vi "RT Driver VI.vi"(7 "Operation":T1, 11 "Device Reference in":T2 format="%.0x") -> (0 "Error Code":i32)   [LabVIEW 2014, in "SLSC configuration Engine.lvlib"]
uses:
  SLSC configuration Engine.lvlib
  <vilib>/NI Veristand/Custom Device API/Custom Device Item Ref.ctl
  <vilib>/NI Veristand/Custom Device API/Hardware Interface Driver VI Operation.ctl
  Type Defs/RT data.ctl
  Type Defs/RT Engine Refs.ctl
  Shared/Type Defs/RT IDs.ctl
  Shared/SPI Utility/Slot #.ctl
  Shared/MCP23S17/Chip Address.ctl
  <vilib>/NI Veristand/Custom Device API/Block Data Reference.ctl
  <vilib>/NI Veristand/Custom Device API/Data Reference.ctl
  <vilib>/FPGAPlugInAG/Dynamic/niLvFpga_Close_Dynamic.vi
  <vilib>/rvi/interface/nirviCloseFPGA/nirviCloseFPGA.xnode
  Shared/SLSC configuration Shared.lvlib
  <vilib>/NI Veristand/Custom Device API/Custom Device API.lvlib
  <vilib>/NI Veristand/Custom Device Tools/Custom Device Utility Library/Custom Device Utility Library.lvlib
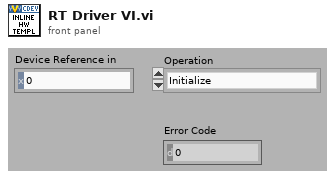
[diagram p1: front panel]
types:
  T1 = typedef "Custom Device API.lvlib/Hardware Interface Driver VI Operation.ctl" = enum16{"Initialize", "Start", "Read Data from HW", "Write Data to HW", "Close"}
  T2 = typedef "Custom Device API.lvlib/Custom Device Item Ref.ctl" = u64
  T3 = typedef "SLSC configuration Engine.lvlib/RT data.ctl" = cluster{"Bitfile ref":refnum<k20>, "Device Error":errorcluster, "FIU Engine Refs":T4, "DMA FIFO ref":refnum<k20>, "Battery Switch Engine Refs":T4, "Wheel Speed Sensor Engine Refs":T4, "Resistor Engine Refs":T4, "Current Sense Engine Refs":T4, "Device Name":string, "LED Engine Refs":T4, "DIO Engine Refs":T4}
  T4 = typedef "SLSC configuration Engine.lvlib/RT Engine Refs.ctl" = cluster{"RT IDs":T5[], "RT Block Data Refs":T8[], "RT Channel Values":dbl[]}
  T5 = typedef "SLSC configuration Shared.lvlib/RT IDs.ctl" = cluster{"Rack #":u8, "Slot #":T6, "Chip Address (A2 A1 A0)":T7}
  T6 = typedef "SLSC configuration Shared.lvlib/Slot #.ctl" = u8
  T7 = typedef "SLSC configuration Shared.lvlib/Chip Address.ctl" = u8
  T8 = typedef "Custom Device API.lvlib/Block Data Reference.ctl" = cluster{"Data Reference":T9, "Offset":i32, "Length":i32}
  T9 = typedef "Custom Device API.lvlib/Data Reference.ctl" = i32
  T10 = typedef "Custom Device API.lvlib/Custom Device Item Info.ctl" = cluster{"Name":string, "Is Channel":bool, "GUID":string, "Is Waveform":bool}
  T11 = typedef "SLSC configuration Shared.lvlib/SLSC compiled.ctl" = cluster{"FIU Engine Data":T12, "Battery Switch Engine Data":T12, "Wheel Speed Sensor Engine Data":T12, "Resistor Engine Data":T12, "Current Sense Engine Data":T12, "LED Engine Data":T12, "DIO Engine Data":T12}
  T12 = typedef "SLSC configuration Shared.lvlib/RT Engine Data.ctl" = cluster{"RT IDs":T5[], "Ordered Channels":T2[]}
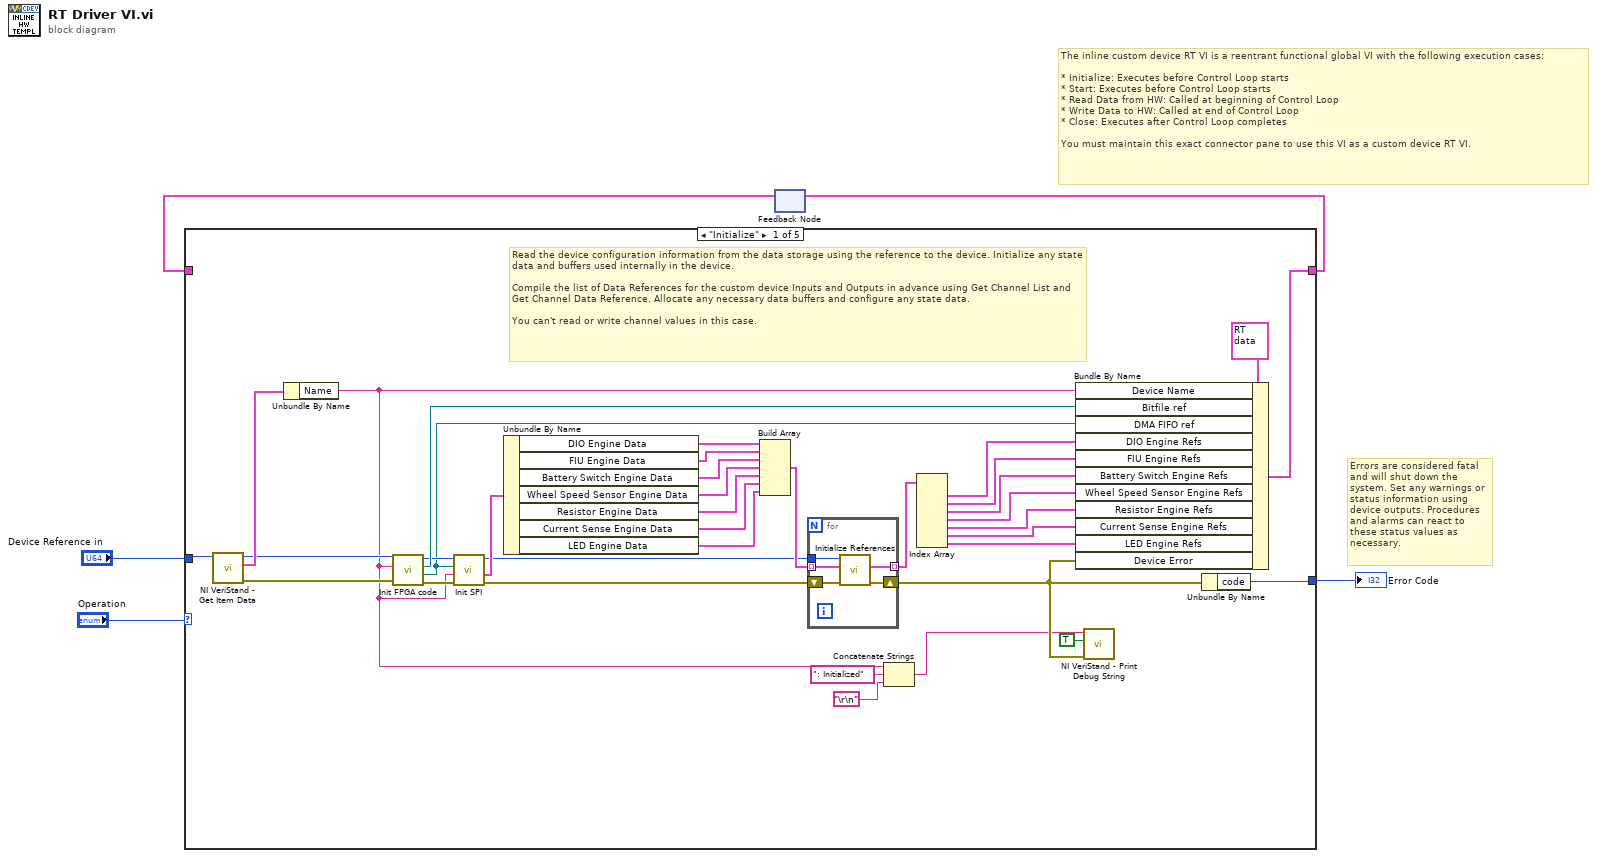
[diagram p0: block diagram]
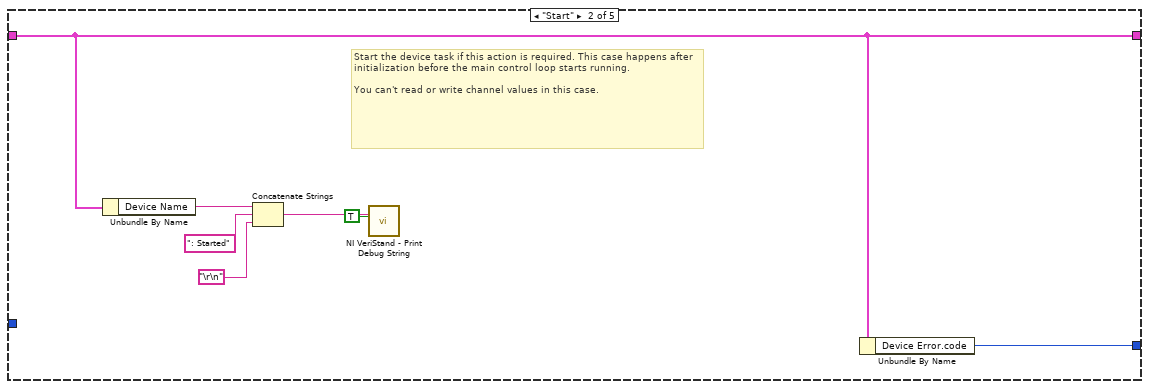
[diagram p2: hidden frame]
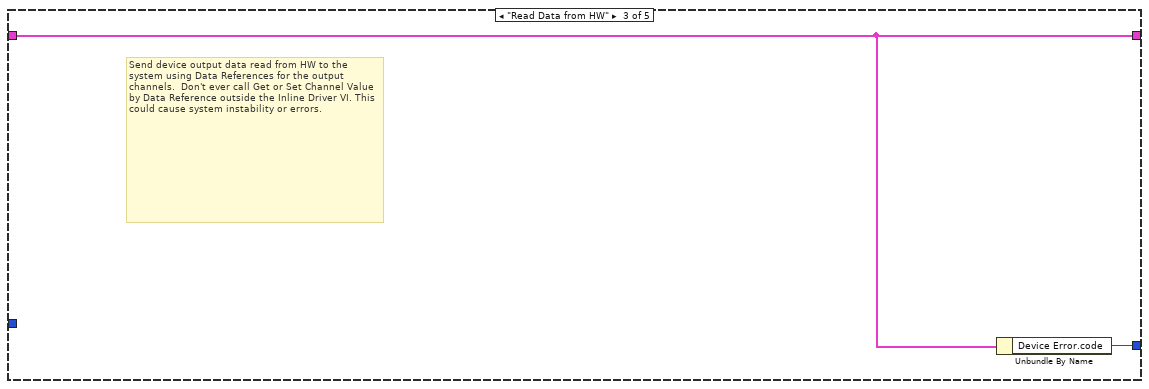
[diagram p3: hidden frame]
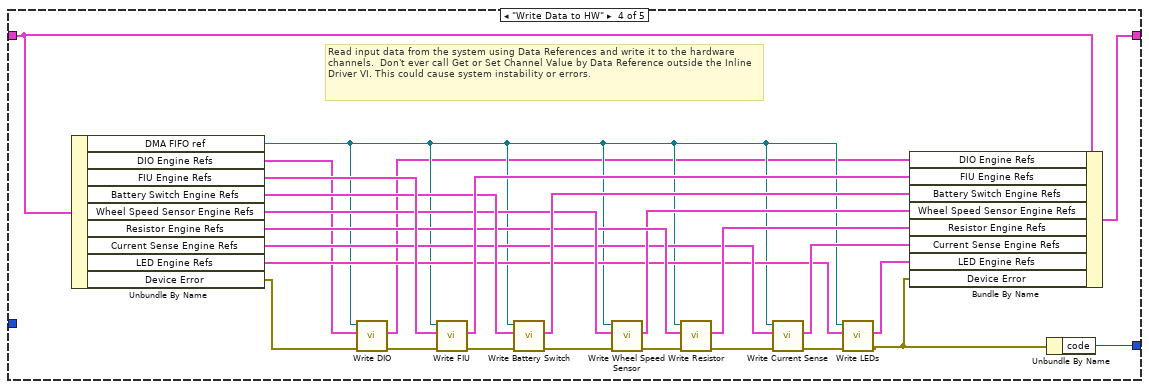
[diagram p4: hidden frame]
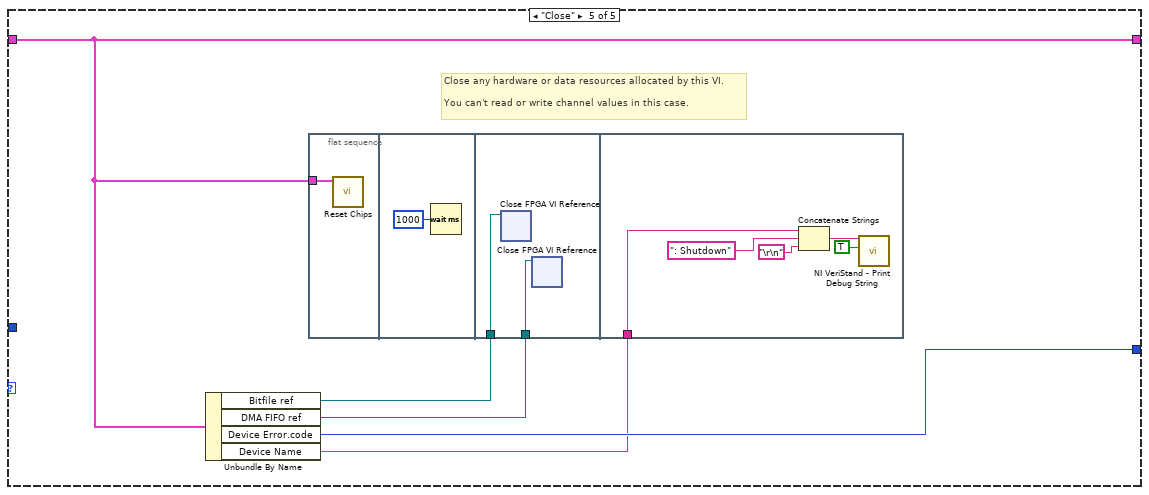
[diagram p5: hidden frame]
diagram:
  # "Errors are considered fatal and will shut down the system. Set any warnings or status information using device outputs. Procedures and alarms can react to these status values as necessary."
  # "The inline custom device RT VI is a reentrant functional global VI with the following execution cases:\n\n* Initialize: Executes before Control Loop starts\n* Start: Executes before Control Loop starts\n* Read Data from HW: Called at beginning of Control Loop\n* Write Data to HW: Called at end of Control Loop\n* Close: Executes after Control Loop completes\n\nYou must maintain this exact connector pane to use this VI as a custom device RT VI."
  n1 = feedback #1() -> (w3:T3)  [unwired: 1 out]
  n2 = case shown="\"Initialize\"" "Operation" {
    tunnel: [w41 w52 w54 w80 w85] -> w4
    tunnel: w3 -> [_ w52 w54 w81 w85]
    tunnel: "Device Reference in" -> [w21 _ _ _ _]
    tunnel: [w40 w53 w55 w79 w86] -> w1
    frame "Initialize" {
      # "Read the device configuration information from the data storage using the reference to the device. Initialize any state data and buffers used internally in the device.\n\nCompile the list of Data References for the custom device Inputs and Outputs in advance using Get Channel List and Get Channel Data Reference. Allocate any necessary data buffers and configure any state data.\n\nYou can't read or write channel values in this case."
      n3 = call <vilib>:"NI VeriStand - Get Item Data.vi"("Item Ref in"=w21) -> ("error out"=w13:errorcluster, "Item Info"=w22:T10, "Item Ref out"=w12:T2)  [unwired: 7 in, 1 out]
      n4 = Unbundle By Name(w22) -> ("Name"=w8:string)
      n5 = call "Init FPGA code.vi"("error in (no error)"=w13, "Name"=w8, "Device Ref in"=w12) -> ("Error out"=w38:errorcluster, "DMA FIFO ref"=w16:refnum<k20>, "Bitfile ref"=w37:refnum<k20>, "Device Ref out"=w36:T2)  [unwired: 5 in]
      n6 = call "Init SPI.vi"("error in (no error)"=w38, "Name"=w8, "DMA FIFO ref in"=w16, "Device Ref in"=w36) -> ("error out"=w11:errorcluster, "Compiled Info"=w25:T11, "Device Ref out"=w9:T2)  [unwired: 5 in]
      n7 = Unbundle By Name(w25) -> ("DIO Engine Data"=w7:T12, "FIU Engine Data"=w35:T12, "Battery Switch Engine Data"=w34:T12, "Wheel Speed Sensor Engine Data"=w30:T12, "Resistor Engine Data"=w28:T12, "Current Sense Engine Data"=w26:T12, "LED Engine Data"=w10:T12)
      n8 = Build Array(w7, w35, w34, w30, w28, w26, w10) -> (w14:T12[])
      n9 = for {
        tunnel: [w44] -> w33 mode=indexing
        shift-right: [w45] -> w23
        shift-left: w11 -> [w46]
        tunnel: w14 -> [w43] mode=indexing
        tunnel: w9 -> [w42]
        n10 = call "Initialize References.vi"("error in (no error)"=w46, "RT Engine Data in"=w43, "Device Ref in"=w42) -> ("error out"=w45:errorcluster, "RT Engine Refs"=w44:T4)  [unwired: 6 in, 1 out]
      }
      n11 = Concatenate Strings(w8, ": Initialized" ("string"), "\r\n") -> (w19:string)
      n12 = Index Array(array=w33) -> (element #1=w6:T4, element #2=w32:T4, element #3=w31:T4, element #4=w29:T4, element #5=w27:T4, element #6=w24:T4, element #7=w15:T4)  [unwired: 7 in]
      n13 = Bundle By Name(cluster=T3 {"Bitfile ref"=refnum, "Device Error"={"status"=FALSE, "code"=0, "source"=""}, "FIU Engine Refs"={"RT IDs"=[], "RT Block Data Refs"=[], "RT Channel Values"=[]}, "DMA FIFO ref"=refnum, "Battery Switch Engine Refs"={"RT IDs"=[], "RT Block Data Refs"=[], "RT Channel Values"=[]}, "Wheel Speed Sensor Engine Refs"={"RT IDs"=[], "RT Block Data Refs"=[], "RT Channel Values"=[]}, "Resistor Engine Refs"={"RT IDs"=[], "RT Block Data Refs"=[], "RT Channel Values"=[]}, "Current Sense Engine Refs"={"RT IDs"=[], "RT Block Data Refs"=[], "RT Channel Values"=[]}, "Device Name"="", "LED Engine Refs"={"RT IDs"=[], "RT Block Data Refs"=[], "RT Channel Values"=[]}, "DIO Engine Refs"={"RT IDs"=[], "RT Block Data Refs"=[], "RT Channel Values"=[]}}, "Device Name"=w8, "Bitfile ref"=w37, "DMA FIFO ref"=w16, "DIO Engine Refs"=w6, "FIU Engine Refs"=w32, "Battery Switch Engine Refs"=w31, "Wheel Speed Sensor Engine Refs"=w29, "Resistor Engine Refs"=w27, "Current Sense Engine Refs"=w24, "LED Engine Refs"=w15, "Device Error"=w23) -> (w41:T3)
      n14 = call <vilib>:"NI VeriStand - Print Debug String.vi"("error in (no error)"=w23, "Add to log file? (T)"=TRUE, "Message"=w19) -> ()  [unwired: 8 in, 1 out]
      n15 = Unbundle By Name(w23) -> ("code"=w40:i32)
    }
    frame "Start" {
      # "Start the device task if this action is required. This case happens after initialization before the main control loop starts running.\n\nYou can't read or write channel values in this case."
      n16 = Unbundle By Name(w52) -> ("Device Name"=w50:string)
      n17 = Concatenate Strings(w50, ": Started" ("string"), "\r\n") -> (w49:string)
      n18 = call <vilib>:"NI VeriStand - Print Debug String.vi"("Add to log file? (T)"=TRUE, "Message"=w49) -> ()  [unwired: 9 in, 1 out]
      n19 = Unbundle By Name(w52) -> ("Device Error.code"=w53:i32)
    }
    frame "Read Data from HW" {
      # "Send device output data read from HW to the system using Data References for the output channels.  Don't ever call Get or Set Channel Value by Data Reference outside the Inline Driver VI. This could cause system instability or errors."
      n20 = Unbundle By Name(w54) -> ("Device Error.code"=w55:i32)
    }
    frame "Write Data to HW" {
      # "Read input data from the system using Data References and write it to the hardware channels.  Don't ever call Get or Set Channel Value by Data Reference outside the Inline Driver VI. This could cause system instability or errors."
      n21 = Unbundle By Name(w81) -> ("DMA FIFO ref"=w59:refnum<k20>, "DIO Engine Refs"=w58:T4, "FIU Engine Refs"=w78:T4, "Battery Switch Engine Refs"=w75:T4, "Wheel Speed Sensor Engine Refs"=w72:T4, "Resistor Engine Refs"=w70:T4, "Current Sense Engine Refs"=w66:T4, "LED Engine Refs"=w63:T4, "Device Error"=w60:errorcluster)
      n22 = call "Write DIO.vi"("error in (no error)"=w60, "FIU Engine Refs in"=w58, "DMA FIFO Ref in"=w59) -> ("error out"=w57:errorcluster, "FIU Engine Refs out"=w56:T4)  [unwired: 7 in]
      n23 = call "Write FIU.vi"("error in (no error)"=w57, "FIU Engine Refs in"=w78, "DMA FIFO Ref in"=w59) -> ("error out"=w76:errorcluster, "FIU Engine Refs out"=w77:T4)  [unwired: 7 in]
      n24 = call "Write Battery Switch.vi"("error in (no error)"=w76, "Battery Switch Engine Refs in"=w75, "DMA FIFO Ref in"=w59) -> ("error out"=w73:errorcluster, "Battery Switch Engine Refs out"=w74:T4)  [unwired: 7 in]
      n25 = call "Write Wheel Speed Sensor.vi"("error in (no error)"=w73, "Wheel Speed Sensor Engine Refs in"=w72, "DMA FIFO Ref in"=w59) -> ("error out"=w71:errorcluster, "Wheel Speed Sensor Engine Refs out"=w68:T4)  [unwired: 7 in]
      n26 = call "Write Resistor.vi"("error in (no error)"=w71, "Resistor Engine Refs in"=w70, "DMA FIFO Ref in"=w59) -> ("error out"=w67:errorcluster, "Resistor Engine Refs out"=w69:T4)  [unwired: 7 in]
      n27 = call "Write Current Sense.vi"("error in (no error)"=w67, "Current Sense Engine Refs in"=w66, "DMA FIFO Ref in"=w59) -> ("error out"=w64:errorcluster, "Current Sense Engine Refs out"=w65:T4)  [unwired: 7 in]
      n28 = call "Write LEDs.vi"("error in (no error)"=w64, "LED Engine Refs in"=w63, "DMA FIFO Ref in"=w59) -> ("error out"=w61:errorcluster, "LED Engine Refs out"=w62:T4)  [unwired: 7 in]
      n29 = Bundle By Name(cluster=w81, "DIO Engine Refs"=w56, "FIU Engine Refs"=w77, "Battery Switch Engine Refs"=w74, "Wheel Speed Sensor Engine Refs"=w68, "Resistor Engine Refs"=w69, "Current Sense Engine Refs"=w65, "LED Engine Refs"=w62, "Device Error"=w61) -> (w80:T3)
      n30 = Unbundle By Name(w61) -> ("code"=w79:i32)
    }
    frame "Close" {
      # "Close any hardware or data resources allocated by this VI.\n\nYou can't read or write channel values in this case."
      n31 = Unbundle By Name(w85) -> ("Bitfile ref"=w84:refnum<k20>, "DMA FIFO ref"=w83:refnum<k20>, "Device Error.code"=w86:i32, "Device Name"=w82:string)
      n32 = flat-sequence {
        tunnel: w85 -> [w87]
        tunnel: w84 -> [w90]
        tunnel: w83 -> [w89]
        tunnel: w82 -> [w91]
        frame #0 {
          n33 = call "Reset Chips.vi"("RT data"=w87) -> ()  [unwired: 10 in, 1 out]
        }
        frame #1 {
          n34 = Wait (ms)(milliseconds to wait=u32 1000) -> ()  [unwired: 1 out]
        }
        frame #2 {
          n35 = xnode "Close FPGA VI Reference"("FPGA VI Reference In"=w90) -> ()  [unwired: 1 in, 1 out]
          n36 = xnode "Close FPGA VI Reference"("FPGA VI Reference In"=w89) -> ()  [unwired: 1 in, 1 out]
        }
        frame #3 {
          n37 = Concatenate Strings(w91, ": Shutdown" ("string"), "\r\n") -> (w93:string)
          n38 = call <vilib>:"NI VeriStand - Print Debug String.vi"("Add to log file? (T)"=TRUE, "Message"=w93) -> ()  [unwired: 9 in, 1 out]
        }
      }
    }
  }
  "Error Code" <- w1
  n39 = feedback-in #1(w4) -> ()
